vi "Periodic Tasks.vi"(8 "error in":errorcluster) -> ()   [LabVIEW 2014]
doc: "This VI runs in parallel to other tasks. It can contain as many user-defined periodic loops as you need. These can carry out PID or other sorts of timed response."
uses:
  <vilib>/Rock Robotics/WPI/DriverStation/WPI_DriverStationRobotMode2.ctl
  <vilib>/Rock Robotics/WPI/Solenoid/WPI_SolenoidValue.ctl
  <vilib>/Rock Robotics/WPI/RobotDrive/WPI_RobotDriveGetSetRefNum.vi
  <vilib>/Rock Robotics/WPI/Joystick/WPI_JoystickGetSetRefNum.vi
  Robot Global Data.vi
  <vilib>/Rock Robotics/Network Tables/SD Write Boolean.vi
  <vilib>/Rock Robotics/Network Tables/SD Write Number.vi
  <vilib>/Rock Robotics/WPI/Compressor/WPI_CompressorGetSetRefNum.vi
  Moose Code/Auto_Conf.vi
  <vilib>/Rock Robotics/WPI/Solenoid/WPI_SolenoidSetEnum.vi
  <vilib>/Rock Robotics/WPI/Solenoid/Deprecated/WPI_SolenoidSetBool.vi
panel:
  in  "Kpd":dbl=0.036
  in  "AllowZero":bool
  in  "ElevatorReset":bool
  out "GoatDetectorPhotoeye":bool
  out "D Contribution":dbl
  in  "Kd":dbl=0.075
  out "BottomOvertravel":bool=TRUE
  out "TopOvertravel":bool=TRUE
  out "ElevatorCurrent":dbl
  out "Voltage":dbl
  out "CurrentSum":dbl
  out "Motor Control":dbl(graph)
  in  "IZone":dbl=25.0
  out "Current":dbl
  out "Target":dbl
  out "PIDPhotoeye":bool
  in  "Kp":dbl=0.036
  in  "Ki":dbl=0.0005 step=0.0001
  out "Target vs. Actual":T1(graph)
  out "I Contribution":dbl
  out "P Contribution":dbl
  in  "Threshold":dbl=3.5
  out "In Position":bool
  out "EncoderLeft":dbl
  out "EncoderRight":dbl
  # "K Tune-torial: (copied from email)\n      Find a P gain that gets you close to your target without overshooting.  \nBased on that P gain value calculate the error at which your P starts to\ndecrease below full throttle.  Make your I cap equal to this error.  Make your\ninitial I gain very small (less than .1 say .0001).  The idea is to accumulate a \nvalue that is manageable. The Talon I accumulates every 1 millisecond so it\nis very easy to calculate the amount of time to get to full throttle.  An I gain\nof .001 will get you full throttle in about 1 second (assuming error never\nchanges).\n      The goal of this strategy is to make I perceivable while still allowing\nP to be the dominating component.  In position servo, I is only needed\nwhen P is not enough to get you to your target.  Once your P output is\nless than full throttle, I will start to kick in.  At first there will be a noticeable\ngap in throttle.  Throttle will decrease proportional to the error and then\nslowly ramp back up until the target is reached, this is useful in observing\nthe effect of I.  Slowly increase I and adjust the I zone until the throttle is \nalmost seamless."
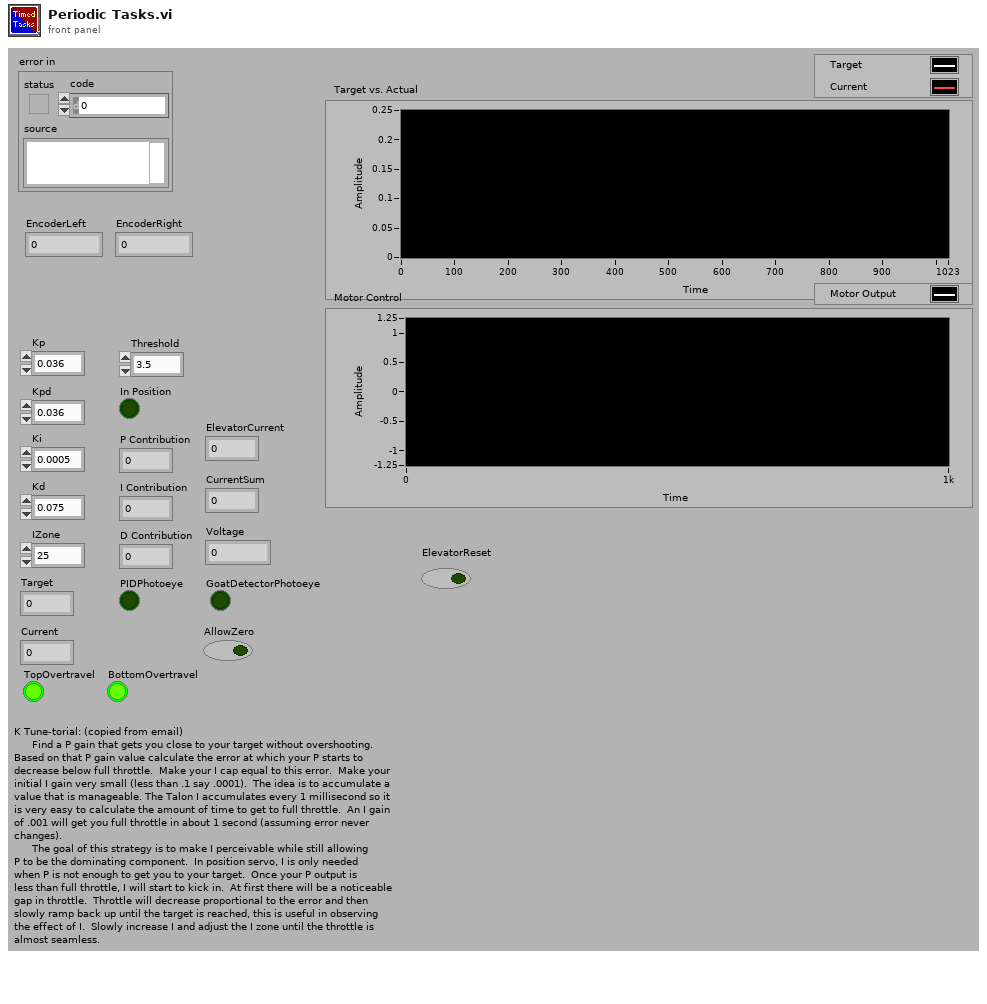
[diagram p1: front panel]
types:
  T1 = cluster{"[0]":dbl, "[1]":dbl, "[2]":dbl, "[3]":dbl, "[4]":dbl, "[5]":dbl, "[6]":dbl, "[7]":dbl, "[8]":dbl}
  T2 = enum16{"ResetForward", "ResetBack", "PIDControl", "ManualControl", "ZeroEncoderAndTarget", "AutoStack"}
  T3 = enum16{"Disabled", "Initialize", "CalcNewTarget", "Moving", "OpenArm", "CloseArm", "Reset"}
  T4 = typedef "WPI_EncoderDevRef.ctl" = cluster{"DevStatus":errorcluster, "EncoderIndex":T5, "CounterIndex":T6, "DistancePerCount":dbl, "Decoding Type":T7}
  T5 = typedef "FPGA_EncoderIdx.ctl" = enum8{"Enc 0", "Enc 1", "Enc 2", "Enc 3", "Enc 4", "Enc 5", "Enc 6", "Enc 7", "Invalid"}
  T6 = typedef "FPGA_CounterCtrSystemIndex.ctl" = enum8{"Ctr 0", "Ctr 1", "Ctr 2", "Ctr 3", "Ctr 4", "Ctr 5", "Ctr 6", "Ctr 7", "Invalid"}
  T7 = typedef "WPI_EncoderType.ctl" = enum16{"1x", "2x", "4x"}
  T8 = typedef "WPI_JoystickDevRef.ctl" = cluster{"Device":T9}
  T9 = typedef "WPI_JoystickDeviceEnum.ctl" = enum16{"USB 0", "USB 1", "USB 2", "USB 3", "USB 4", "USB 5"}
  T10 = typedef "WPI_SolenoidDevRef.ctl" = cluster{"DevStatus":errorcluster, "Pneumatics Control Module":u8, "Forward Solenoid Channel":T11, "Reverse Solenoid Channel":T11}
  T11 = typedef "WPI_SolenoidChannel.ctl" = enum8{"Solenoid 0", "Solenoid 1", "Solenoid 2", "Solenoid 3", "Solenoid 4", "Solenoid 5", "Solenoid 6", "Solenoid 7", "Invalid"}
  T12 = typedef "WPI_MotorControlDeviceRef.ctl" = cluster{"DeviceStatus":errorcluster, "Type":T13, "PWM":cluster{"Controller":T14, "PWM Channel":T15, "DeadBand":T16}, "CAN":cluster{"Device Number":u8, "Control Mode":T17, "Semaphore":T18, "Max Vout":dbl, "TalonSRX Control Mode":T19}, "Invert":bool, "TransformRef":T20, "InvTransformRef":T20}
  T13 = typedef "WPI_MotorControlType.ctl" = enum16{"PWM", "CAN", "CANTalonSRX"}
  T14 = typedef "FPGA_TypedefDigitalModule.ctl" = enum16{"Controller 1"}
  T15 = typedef "FPGA_DIOPWMChannel.ctl" = enum8{"PWM 0", "PWM 1", "PWM 2", "PWM 3", "PWM 4", "PWM 5", "PWM 6", "PWM 7", "PWM 8", "PWM 9", "PWM MXP 0", "PWM MXP 1", "PWM MXP 2", "PWM MXP 3", "PWM MXP 4", "PWM MXP 5", "PWM MXP 6", "PWM MXP 7", "PWM MXP 8", "PWM MXP 9", "Invalid"}
  T16 = typedef "WPI_PWMDeadband.ctl" = cluster{"Name":string, "maxPositivePwm":i32, "minPositivePwm":i32, "centerPwm":i32, "maxNegativePwm":i32, "minNegativePwm":i32, "angularRange":u16}
  T17 = typedef "WPI_CANJaguar_ControlMode.ctl" = enum8{"Percent VBus", "Current", "Speed", "Position", "Voltage"}
  T18 = typedef "Semaphore RefNum" = refnum<k1>
  T19 = typedef "WPI_CANTalonSRX_APIControlMode.ctl" = enum8{"Percent VBus", "Speed", "Position", "Slave", "Unchanged / Invalid"}
  T20 = typedef "WPI_PWMTransform_ConPane.ctl" = refnum<vi>
  T21 = typedef "WPI_RobotDriveDevRef.ctl" = cluster{"DevStatus":errorcluster, "Motors[]":T12[], "Square Inputs":bool, "Max Output":dbl}
  T22 = typedef "WPI_DigitalInputDevRef.ctl" = cluster{"DevStatus":errorcluster, "DIO Channel":T23, "Controller":T14}
  T23 = typedef "FPGA_DIOChannel.ctl" = enum8{"DIO 0", "DIO 1", "DIO 2", "DIO 3", "DIO 4", "DIO 5", "DIO 6", "DIO 7", "DIO 8", "DIO 9", "DIO MXP 0", "DIO MXP 1", "DIO MXP 2", "DIO MXP 3", "DIO MXP 4", "DIO MXP 5", "DIO MXP 6", "DIO MXP 7", "DIO MXP 8", "DIO MXP 9", "DIO MXP 10", "DIO MXP 11", "DIO MXP 12", "DIO MXP 13", "DIO MXP 14", "DIO MXP 15", "Invalid"}
  T24 = typedef "WPI_CompressorDevRef.ctl" = cluster{"DevStatus":errorcluster, "Pneumatics Control Module":u8}
  T25 = typedef "WPI_DriverStationRobotMode2.ctl" = enum16{"Autonomous Disabled", "Autonomous Enabled", "Teleop Disabled", "Teleop Enabled", "Disconnected", "Finish", "Test Disabled", "Test Enabled", "Emergency Stopped"}
  T26 = typedef "WPI_GyroDevRef.ctl" = cluster{"DevStatus":errorcluster, "Analog Module":T27, "Analog Channel":T28, "Offset":dbl, "Gain (VoltsPerDegree/Second)":dbl}
  T27 = typedef "FPGA_TypedefAnalogModule.ctl" = enum16{"Controller 1"}
  T28 = typedef "FPGA_AIChannel.ctl" = enum8{"AI 0", "AI 1", "AI 2", "AI 3", "AI MXP 0", "AI MXP 1", "AI MXP 2", "AI MXP 3", "Invalid"}
  T29 = typedef "WPI_SolenoidValue.ctl" = enum16{"Off", "On", "Forward", "Reverse"}
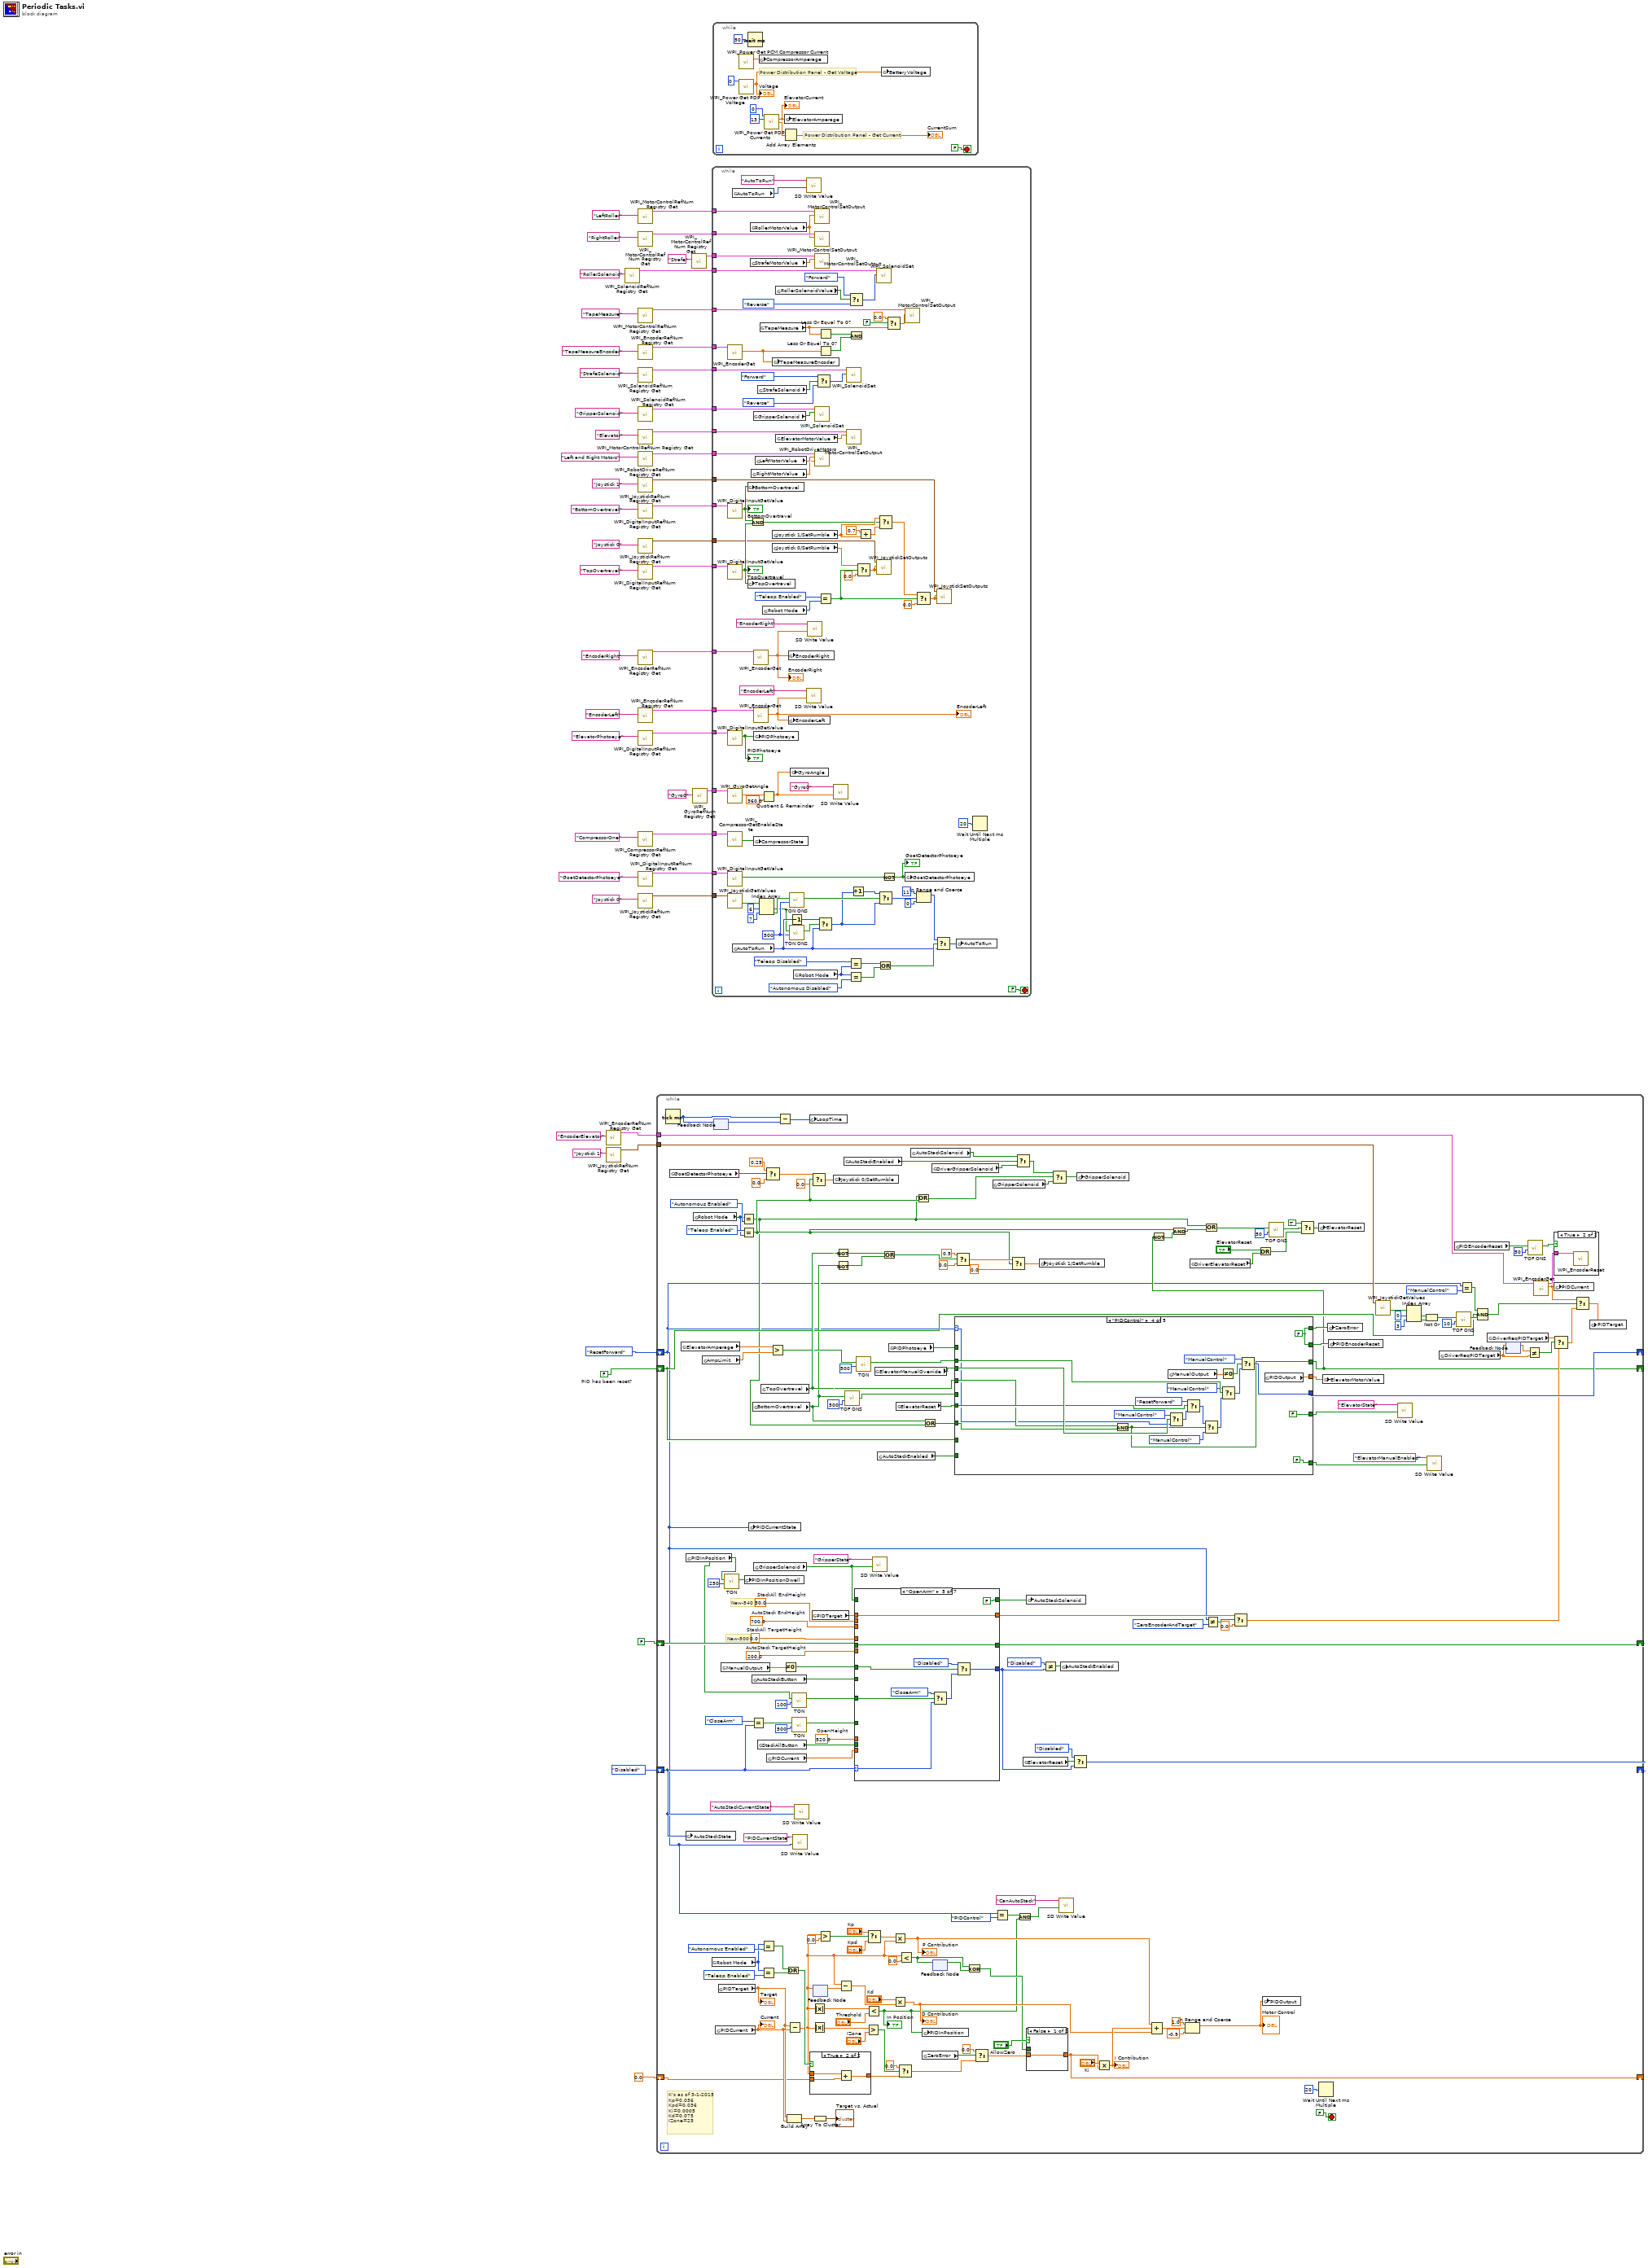
[diagram p0: block diagram]
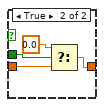
[diagram p4: hidden frame]
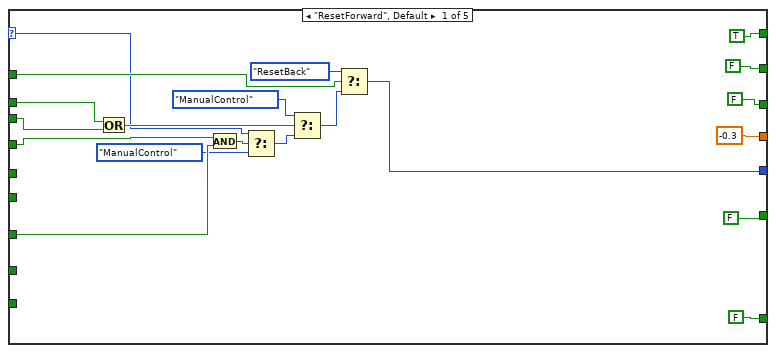
[diagram p5: hidden frame]
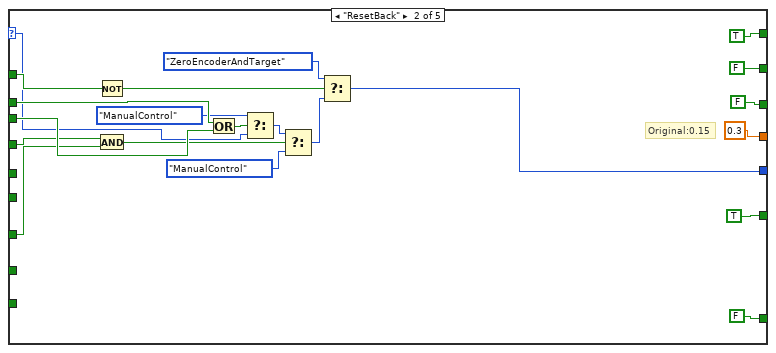
[diagram p6: hidden frame]
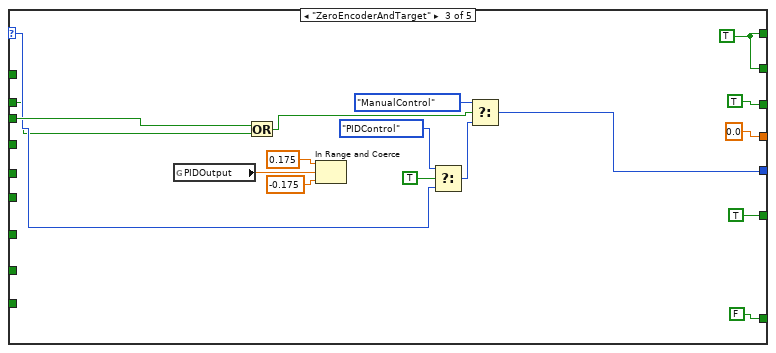
[diagram p7: hidden frame]
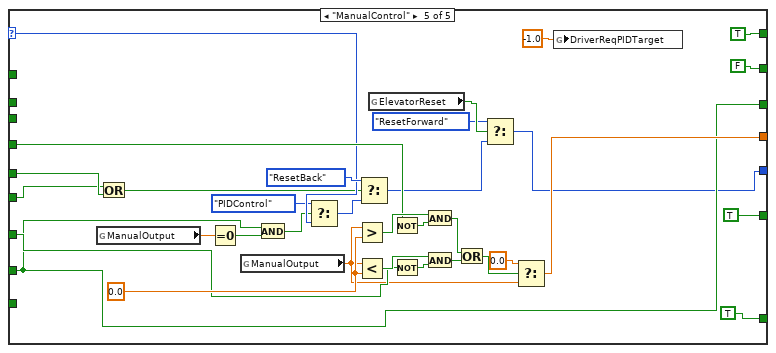
[diagram p8: hidden frame]
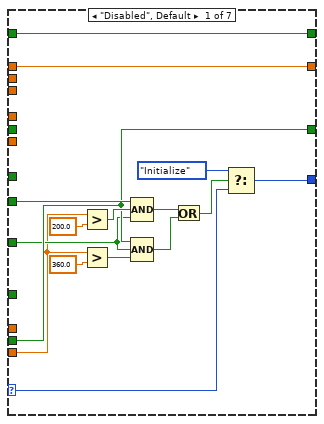
[diagram p9: hidden frame]
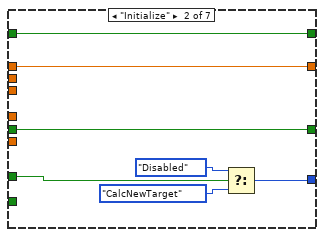
[diagram p10: hidden frame]
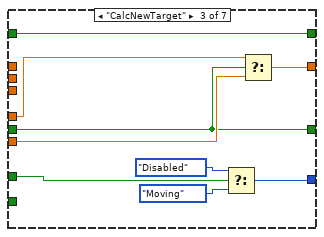
[diagram p11: hidden frame]
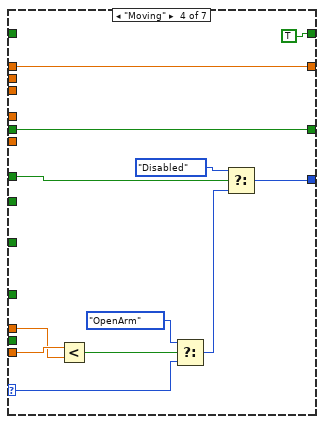
[diagram p12: hidden frame]
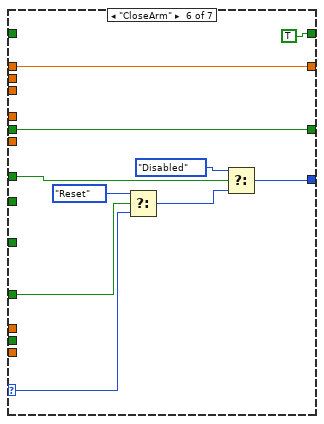
[diagram p13: hidden frame]
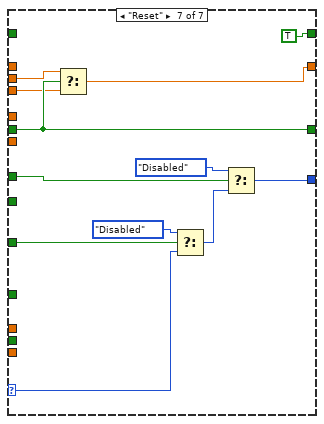
[diagram p14: hidden frame]
diagram:
  w20 = FALSE  # PID has been reset?
  n1 = call <vilib>:"WPI_EncoderRefNum Registry Get.vi"("refnum name"="EncoderElevator") -> ("EncoderDevRef"=w9:T4)  [unwired: 9 in, 1 out]
  n2 = call <vilib>:"WPI_JoystickRefNum Registry Get.vi"("refnum name"="Joystick 1") -> ("JoystickDevRef"=w7:T8)  [unwired: 9 in, 1 out]
  n3 = call <vilib>:"WPI_SolenoidRefNum Registry Get.vi"("refnum name"="RollerSolenoid") -> ("SolenoidDevRef"=w10:T10)  [unwired: 9 in, 1 out]
  n4 = call <vilib>:"WPI_MotorControlRefNum Registry Get.vi"("refnum name"="LeftRoller") -> ("MotorControlDevRef"=w13:T12)  [unwired: 9 in, 1 out]
  n5 = call <vilib>:"WPI_MotorControlRefNum Registry Get.vi"("refnum name"="RightRoller") -> ("MotorControlDevRef"=w12:T12)  [unwired: 9 in, 1 out]
  n6 = call <vilib>:"WPI_MotorControlRefNum Registry Get.vi"("refnum name"="TapeMeasure") -> ("MotorControlDevRef"=w4:T12)  [unwired: 9 in, 1 out]
  n7 = call <vilib>:"WPI_EncoderRefNum Registry Get.vi"("refnum name"="TapeMeasureEncoder") -> ("EncoderDevRef"=w1:T4)  [unwired: 9 in, 1 out]
  n8 = call <vilib>:"WPI_SolenoidRefNum Registry Get.vi"("refnum name"="StrafeSolenoid") -> ("SolenoidDevRef"=w16:T10)  [unwired: 9 in, 1 out]
  n9 = call <vilib>:"WPI_SolenoidRefNum Registry Get.vi"("refnum name"="GripperSolenoid") -> ("SolenoidDevRef"=w30:T10)  [unwired: 9 in, 1 out]
  n10 = call <vilib>:"WPI_MotorControlRefNum Registry Get.vi"("refnum name"="Elevator") -> ("MotorControlDevRef"=w46:T12)  [unwired: 9 in, 1 out]
  n11 = call <vilib>:"WPI_RobotDriveRefNum Registry Get.vi"("refnum name"="Left and Right Motors") -> ("RobotDriveDevRef"=w51:T21)  [unwired: 9 in, 1 out]
  n12 = call <vilib>:"WPI_JoystickRefNum Registry Get.vi"("refnum name"="Joystick 1") -> ("JoystickDevRef"=w27:T8)  [unwired: 1 in, 9 out]
  n13 = call <vilib>:"WPI_DigitalInputRefNum Registry Get.vi"("refnum name"="BottomOvertravel") -> ("DigitalInputDevRef"=w32:T22)  [unwired: 9 in, 1 out]
  n14 = call <vilib>:"WPI_JoystickRefNum Registry Get.vi"("refnum name"="Joystick 0") -> ("JoystickDevRef"=w26:T8)  [unwired: 1 in, 9 out]
  n15 = call <vilib>:"WPI_DigitalInputRefNum Registry Get.vi"("refnum name"="TopOvertravel") -> ("DigitalInputDevRef"=w34:T22)  [unwired: 9 in, 1 out]
  n16 = call <vilib>:"WPI_EncoderRefNum Registry Get.vi"("refnum name"="EncoderRight") -> ("EncoderDevRef"=w39:T4)  [unwired: 9 in, 1 out]
  n17 = call <vilib>:"WPI_EncoderRefNum Registry Get.vi"("refnum name"="EncoderLeft") -> ("EncoderDevRef"=w41:T4)  [unwired: 9 in, 1 out]
  n18 = call <vilib>:"WPI_DigitalInputRefNum Registry Get.vi"("refnum name"="ElevatorPhotoeye") -> ("DigitalInputDevRef"=w44:T22)  [unwired: 9 in, 1 out]
  n19 = call <vilib>:"WPI_CompressorRefNum Registry Get.vi"("refnum name"="CompressorOne") -> ("CompressorDevRef"=w5:T24)  [unwired: 9 in, 1 out]
  n20 = call <vilib>:"WPI_DigitalInputRefNum Registry Get.vi"("refnum name"="GoatDetectorPhotoeye") -> ("DigitalInputDevRef"=w24:T22)  [unwired: 9 in, 1 out]
  n21 = call <vilib>:"WPI_JoystickRefNum Registry Get.vi"("refnum name"="Joystick 0") -> ("JoystickDevRef"=w18:T8)  [unwired: 9 in, 1 out]
  n22 = while {
    shift-right: [w136] -> _
    shift-left: 0.0 -> [w65]
    shift-right: [w126] -> _
    shift-left: T3."Disabled" -> [w102]
    shift-right: [w202] -> _
    shift-left: FALSE -> [w204]
    shift-right: [w164] -> _
    shift-left: T2."ResetForward" -> [w56]
    shift-right: [w58] -> _
    shift-left: w20 -> [w109]
    tunnel: w9 -> [w96]
    tunnel: w7 -> [w92]
    stop <- FALSE stop-if-true
    w52 = 0.0  # StackAll TargetHeight
    w82 = 700.0  # AutoStack EndHeight
    w112 = 200.0  # AutoStack TargetHeight
    w113 = 30.0  # StackAll EndHeight
    w205 = 520.0  # OpenHeight
    # "New-500"
    # "New-540"
    # "K's as of 3-1-2015\nKp=0.036\nKpd=0.036\nKi=0.0005\nKd=0.075\nIZone=25"
    n23 = Tick Count (ms)() -> (millisecond timer value=w145:u32)
    n24 = global read "Robot Global Data.vi" "GoatDetectorPhotoeye"() -> (w197:bool)
    n25 = global read "Robot Global Data.vi" "ElevatorAmperage"() -> (w175:dbl)
    n26 = global write "Robot Global Data.vi" "AutoStackState"(w102) -> ()
    n27 = global read "Robot Global Data.vi" "PIDInPosition"() -> (w64:bool)
    n28 = global read "Robot Global Data.vi" "Robot Mode"() -> (w59:T25)
    n29 = global read "Robot Global Data.vi" "AmpLimit"() -> (w176:dbl)
    n30 = global read "Robot Global Data.vi" "Robot Mode"() -> (w69:T25)
    n31 = feedback-in #1(w145) -> ()
    n32 = feedback #1() -> (w144:u32)  [unwired: 1 in]
    n33 = global read "Robot Global Data.vi" "PIDCurrent"() -> (w220:dbl)
    "Current" <- w220
    n34 = global read "Robot Global Data.vi" "PIDTarget"() -> (w216:dbl)
    "Target" <- w216
    n35 = global read "Robot Global Data.vi" "ManualOutput"() -> (w111:dbl)
    n36 = call "TON.vi"("Delay (ms)"=u32 250, "Input"=w64) -> ("Output"=w105:bool)  [unwired: 9 in]
    n37 = Equal?(x=w59, y=WPI_DriverStationRobotMode2."Autonomous Enabled") -> (x = y?=w75:bool)
    n38 = Equal?(x=WPI_DriverStationRobotMode2."Teleop Enabled" ("y"), y=w59) -> (x = y?=w77:bool)
    n39 = global write "Robot Global Data.vi" "PIDInPositionDwell"(w105) -> ()
    n40 = global write "Robot Global Data.vi" "PIDCurrentState"(w56) -> ()
    n41 = Equal?(x=T3."CloseArm" ("t"), y=w102) -> (x = y?=w121:bool)
    n42 = global read "Robot Global Data.vi" "AutoStackButton"() -> (w206:bool)
    n43 = global read "Robot Global Data.vi" "BottomOvertravel"() -> (w84:bool)
    n44 = global read "Robot Global Data.vi" "GripperSolenoid"() -> (w87:bool)
    n45 = global read "Robot Global Data.vi" "StackAllButton"() -> (w208:bool)
    n46 = global read "Robot Global Data.vi" "TopOvertravel"() -> (w194:bool)
    n47 = Equal?(x=w69, y=WPI_DriverStationRobotMode2."Autonomous Enabled") -> (x = y?=w73:bool)
    n48 = Equal?(x=w69, y=WPI_DriverStationRobotMode2."Teleop Enabled") -> (x = y?=w72:bool)
    n49 = Select(t=0.25, s=w197, f=0.0) -> (s? t:f=w195:dbl)
    n50 = global read "Robot Global Data.vi" "PIDCurrent"() -> (w203:dbl)
    n51 = Greater?(x=w175, y=w176) -> (0:w177:bool)
    n52 = Subtract(x=w145, y=w144) -> (x-y=w143:u32)
    n53 = Not Equal To 0?(x=w111) -> (x != 0?=w110:bool)
    n54 = Or(x=w73, y=w72) -> (x .or. y?=w68:bool)
    n55 = Build Array(w216, w220) -> (w224:dbl[])
    n56 = Subtract(x=w216, y=w220) -> (x-y=w66:dbl)
    n57 = call "TON.vi"("Delay (ms)"=u32 100, "Input"=w64) -> ("Output"=w81:bool)  [unwired: 9 in]
    n58 = call "TON.vi"("Delay (ms)"=u32 500, "Input"=w121) -> ("Output"=w123:bool)  [unwired: 9 in]
    n59 = call-poly <vilib>:"SD Write Value.vi"("Numeric"=w56, "Name"="PIDCurrentState") -> ()  [unwired: 8 in, 2 out]
    n60 = call-poly <vilib>:"SD Write Value.vi"("Numeric"=w102, "Name"="AutoStackCurrentState") -> ()  [unwired: 8 in, 2 out]
    n61 = global write "Robot Global Data.vi" "LoopTime"(w143) -> ()
    n62 = case shown="True" w68 {
      tunnel: [w231 w234] -> w67
      tunnel: w66 -> [_ w233]
      tunnel: w65 -> [w231 w232]
      frame False {
      }
      frame True {
        n63 = Add(x=w233, y=w232) -> (x+y=w234:dbl)
      }
    }
    n64 = Select(t=w195, s=w77, f=0.0) -> (s? t:f=w180:dbl)
    n65 = global read "Robot Global Data.vi" "PIDTarget"() -> (w207:dbl)
    n66 = Absolute Value(x=w66) -> (abs(x)=w222:dbl)
    n67 = Absolute Value(x=w66) -> (abs(x)=w219:dbl)
    n68 = feedback-in #2(w66) -> ()
    n69 = feedback #2() -> (w215:dbl)  [unwired: 1 in]
    n70 = Array To Cluster(array=w224) -> (cluster=→"Target vs. Actual":T1)
    n71 = Greater?(x=w66, y=0.0) -> (0:w118:bool)
    n72 = global write "Robot Global Data.vi" "Joystick 0/SetRumble"(w180) -> ()
    n73 = Not(x=w194) -> (.not. x?=w192:bool)
    n74 = Not(x=w84) -> (.not. x?=w193:bool)
    n75 = Subtract(x=w66, y=w215) -> (x-y=w213:dbl)
    n76 = global read "Robot Global Data.vi" "AutoStackEnabled"() -> (w63:bool)
    n77 = call "TOF ONS.vi"("Delay (ms)"=u32 500, "Input"=w84) -> ("Output"=w107:bool)  [unwired: 9 in]
    n78 = case shown="\"OpenArm\"" w102 {
      selector: w102 -> [w370 _ _ w397 w405 w414 w428]
      tunnel: w205 -> [_ _ _ w387 _ _ _]
      tunnel: w112 -> [_ _ w384 _ _ _ _]
      tunnel: w206 -> [w361 _ _ _ _ _ _]
      tunnel: w207 -> [w355 w377 _ w394 w406 w416 _]
      tunnel: [w355 w377 w386 w394 w406 w416 w426] -> w161
      tunnel: w208 -> [w360 _ _ _ _ _ _]
      tunnel: [w360 w376 w379 w393 w408 w417 w425] -> w202
      tunnel: w204 -> [_ w376 w379 w393 w408 w417 w425]
      tunnel: [w366 w375 w385 TRUE FALSE ("Solenoid") TRUE ("Solenoid") TRUE ("Solenoid")] -> w209
      tunnel: w87 -> [w366 w375 w385 _ _ _ _]
      tunnel: [w368 w372 w381 w392 w402 w411 w422] -> w127
      tunnel: w81 -> [w358 _ _ _ w403 _ w429]
      tunnel: w203 -> [w356 _ _ w388 _ _ _]
      tunnel: w123 -> [_ _ _ _ _ w413 _]
      tunnel: w113 -> [_ _ _ _ _ _ w424]
      tunnel: w110 -> [_ w371 w380 w390 w399 w409 w421]
      tunnel: w82 -> [_ _ _ _ _ _ w419]
      tunnel: w52 -> [_ _ w378 _ _ _ _]
      frame "Disabled", Default {
        n79 = Greater?(x=w356, y=200.0) -> (0:w367:bool)
        n80 = Greater?(x=w356, y=360.0) -> (0:w357:bool)
        n81 = Compound Arithmetic op=AND(w361, w367, w358) -> (w364:bool)
        n82 = Compound Arithmetic op=AND(w360, w358, w357) -> (w362:bool)
        n83 = Or(x=w364, y=w362) -> (x .or. y?=w363:bool)
        n84 = Select(t=T3."Initialize", s=w363, f=w370) -> (s? t:f=w368:T3)
      }
      frame "Initialize" {
        n85 = Select(t=T3."Disabled", s=w371, f=T3."CalcNewTarget") -> (s? t:f=w372:T3)
      }
      frame "CalcNewTarget" {
        n86 = Select(t=T3."Disabled", s=w380, f=T3."Moving") -> (s? t:f=w381:T3)
        n87 = Select(t=w378, s=w379, f=w384) -> (s? t:f=w386:dbl)
      }
      frame "Moving" {
        n88 = Less?(x=w388, y=w387) -> (x < y?=w398:bool)
        n89 = Select(t=T3."OpenArm", s=w398, f=w397) -> (s? t:f=w391:T3)
        n90 = Select(t=T3."Disabled", s=w390, f=w391) -> (s? t:f=w392:T3)
      }
      frame "OpenArm" {
        n91 = Select(t=T3."CloseArm", s=w403, f=w405) -> (s? t:f=w401:T3)
        n92 = Select(t=T3."Disabled", s=w399, f=w401) -> (s? t:f=w402:T3)
      }
      frame "CloseArm" {
        n93 = Select(t=T3."Reset", s=w413, f=w414) -> (s? t:f=w410:T3)
        n94 = Select(t=T3."Disabled", s=w409, f=w410) -> (s? t:f=w411:T3)
      }
      frame "Reset" {
        n95 = Select(t=w424, s=w425, f=w419) -> (s? t:f=w426:dbl)
        n96 = Select(t=T3."Disabled", s=w429, f=w428) -> (s? t:f=w420:T3)
        n97 = Select(t=T3."Disabled", s=w421, f=w420) -> (s? t:f=w422:T3)
      }
    }
    n98 = call "TON.vi"("Delay (ms)"=u32 500, "Input"=w177) -> ("Output"=w178:bool)  [unwired: 9 in]
    n99 = Greater?(x=w219, y="IZone") -> (0:w155:bool)
    n100 = Select(t="Kp", s=w118, f="Kpd") -> (s? t:f=w117:dbl)
    n101 = Less?(x=w222, y="Threshold") -> (x < y?=w54:bool)
    "In Position" <- w54
    n102 = call-poly <vilib>:"SD Write Value.vi"("Boolean"=w87, "Name"="GripperState") -> ()  [unwired: 8 in, 2 out]
    n103 = global read "Robot Global Data.vi" "ElevatorManualOverride"() -> (w169:bool)
    n104 = global read "Robot Global Data.vi" "AutoStackEnabled"() -> (w62:bool)
    n105 = Or(x=w192, y=w193) -> (x .or. y?=w190:bool)
    n106 = global read "Robot Global Data.vi" "PIDPhotoeye"() -> (w168:bool)
    n107 = Multiply(x=w117, y=w66) -> (x*y=w156:dbl)
    "P Contribution" <- w156
    n108 = Multiply(x="Kd", y=w213) -> (x*y=w212:dbl)
    "D Contribution" <- w212
    n109 = global read "Robot Global Data.vi" "ElevatorReset"() -> (w170:bool)
    n110 = Select(t=0.0, s=w155, f=w67) -> (s? t:f=w130:dbl)
    n111 = Less?(x=w66, y=0.0) -> (x < y?=w139:bool)
    n112 = global read "Robot Global Data.vi" "AutoStackSolenoid"() -> (w184:bool)
    n113 = Or(x=w75, y=w77) -> (x .or. y?=w186:bool)
    n114 = global write "Robot Global Data.vi" "PIDInPosition"(w54) -> ()
    n115 = global read "Robot Global Data.vi" "ZeroError"() -> (w132:bool)
    n116 = Or(x=w84, y=w75) -> (x .or. y?=w83:bool)
    n117 = global read "Robot Global Data.vi" "DriverGripperSolenoid"() -> (w183:bool)
    n118 = feedback-in #3(w139) -> ()
    n119 = feedback #3() -> (w138:bool)  [unwired: 1 in]
    n120 = case shown="\"PIDControl\"" w56 {
      selector: w56 -> [w242 w263 w293 w302 w334]
      tunnel: [-0.3 0.3 0.0 ("ManualOutput") w301 w353] -> w167
      tunnel: [w244 w264 w298 w306 w323] -> w164
      tunnel: w168 -> [w259 w280 _ _ _]
      tunnel: w169 -> [w246 w278 w297 w321 _]
      tunnel: w170 -> [_ _ _ w320 w329]
      tunnel: [FALSE ("PIDEncoderReset") FALSE ("PIDEncoderReset") w289 w318 FALSE ("PIDEncoderReset")] -> w174
      tunnel: [TRUE ("PIDEncoderReset") TRUE ("PIDEncoderReset") w289 w318 TRUE ("PIDEncoderReset")] -> w79
      tunnel: w194 -> [w256 w274 _ w315 w351]
      tunnel: w83 -> [w255 w273 _ w314 w345]
      tunnel: w178 -> [w248 w270 w287 w313 _]
      tunnel: [FALSE ("PIDEncoderReset") FALSE ("PIDEncoderReset") FALSE ("PIDEncoderReset") FALSE ("PIDEncoderReset") TRUE ("PIDEncoderReset")] -> w151
      tunnel: w62 -> [_ _ _ _ _]
      tunnel: w109 -> [_ _ _ _ w331]
      tunnel: [FALSE FALSE TRUE w299 w331] -> w58
      tunnel: w107 -> [_ _ _ _ w330]
      tunnel: [FALSE ("PIDEncoderReset") TRUE ("PIDEncoderReset") TRUE ("PIDEncoderReset") FALSE ("PIDEncoderReset") TRUE ("PIDEncoderReset")] -> w85
      frame "ResetForward", Default {
        n121 = Or(x=w248, y=w246) -> (x .or. y?=w247:bool)
        n122 = And(x=w256, y=w255) -> (x .and. y?=w257:bool)
        n123 = Select(t=w242, s=w257, f=T2."ManualControl") -> (s? t:f=w252:T2)
        n124 = Select(t=T2."ManualControl", s=w247, f=w252) -> (s? t:f=w243:T2)
        n125 = Select(t=T2."ResetBack", s=w259, f=w243) -> (s? t:f=w244:T2)
      }
      frame "ResetBack" {
        # "Original:0.15"
        n126 = Not(x=w280) -> (.not. x?=w279:bool)
        n127 = And(x=w274, y=w273) -> (x .and. y?=w276:bool)
        n128 = Or(x=w270, y=w278) -> (x .or. y?=w271:bool)
        n129 = Select(t=T2."ManualControl", s=w271, f=w263) -> (s? t:f=w275:T2)
        n130 = Select(t=w275, s=w276, f=T2."ManualControl") -> (s? t:f=w262:T2)
        n131 = Select(t=T2."ZeroEncoderAndTarget", s=w279, f=w262) -> (s? t:f=w264:T2)
      }
      frame "ZeroEncoderAndTarget" {
        w289 = TRUE ("PIDEncoderReset")
        n132 = global read "Robot Global Data.vi" "PIDOutput"() -> (w292:dbl)
        n133 = Or(x=w297, y=w287) -> (x .or. y?=w288:bool)
        n134 = In Range and Coerce(upper limit=0.175, x=w292, lower limit=-0.175) -> ()  [unwired: 2 out]
        n135 = Select(t=T2."PIDControl", s=TRUE, f=w293) -> (s? t:f=w295:T2)
        n136 = Select(t=T2."ManualControl", s=w288, f=w295) -> (s? t:f=w298:T2)
      }
      frame "PIDControl" {
        w318 = FALSE ("PIDEncoderReset")
        n137 = And(x=w315, y=w314) -> (x .and. y?=w299:bool)
        n138 = global read "Robot Global Data.vi" "ManualOutput"() -> (w304:dbl)
        n139 = Select(t=T2."ManualControl", s=w321, f=w302) -> (s? t:f=w319:T2)
        n140 = Select(t=T2."ResetForward", s=w320, f=w319) -> (s? t:f=w316:T2)
        n141 = Select(t=w316, s=w299, f=T2."ManualControl") -> (s? t:f=w317:T2)
        n142 = Not Equal To 0?(x=w304) -> (x != 0?=w303:bool)
        n143 = Select(t=T2."ManualControl", s=w313, f=w317) -> (s? t:f=w307:T2)
        n144 = Select(t=T2."ManualControl", s=w303, f=w307) -> (s? t:f=w306:T2)
        n145 = global read "Robot Global Data.vi" "PIDOutput"() -> (w301:dbl)
      }
      frame "ManualControl" {
        w347 = 0.0 ("y")
        n146 = global read "Robot Global Data.vi" "ManualOutput"() -> (w337:dbl)
        n147 = Or(x=w329, y=w330) -> (x .or. y?=w328:bool)
        n148 = Equal To 0?(x=w337) -> (x = 0?=w336:bool)
        n149 = global read "Robot Global Data.vi" "ManualOutput"() -> (w343:dbl)
        n150 = And(x=w331, y=w336) -> (x .and. y?=w332:bool)
        n151 = Select(t=T2."PIDControl", s=w332, f=w334) -> (s? t:f=w335:T2)
        n152 = Greater?(x=w343, y=w347) -> (0:w352:bool)
        n153 = Less?(x=w343, y=w347) -> (x < y?=w346:bool)
        n154 = Select(t=T2."ResetBack", s=w328, f=w335) -> (s? t:f=w324:T2)
        n155 = global read "Robot Global Data.vi" "ElevatorReset"() -> (w325:bool)
        n156 = Not(x=w351) -> (.not. x?=w341:bool)
        n157 = Not(x=w345) -> (.not. x?=w342:bool)
        n158 = And(x=w352, y=w341) -> (x .and. y?=w349:bool)
        n159 = And(x=w346, y=w342) -> (x .and. y?=w344:bool)
        n160 = Or(x=w349, y=w344) -> (x .or. y?=w348:bool)
        n161 = Select(t=T2."ResetForward", s=w325, f=w324) -> (s? t:f=w323:T2)
        n162 = Select(t=0.0, s=w348, f=w343) -> (s? t:f=w353:dbl)
        n163 = global write "Robot Global Data.vi" "DriverReqPIDTarget"(-1.0 ("DriverReqPIDTarget")) -> ()
      }
    }
    n164 = Select(t=0.5, s=w190, f=0.0) -> (s? t:f=w189:dbl)
    n165 = Exclusive Or(1:w138, 2:w139) -> (0:w135:bool)
    n166 = Select(t=0.0, s=w132, f=w130) -> (s? t:f=w133:dbl)
    n167 = global read "Robot Global Data.vi" "GripperSolenoid"() -> (w187:bool)
    n168 = Equal?(x=w56, y=T2."PIDControl") -> (x = y?=w55:bool)
    n169 = Select(t=w189, s=w77, f=0.0) -> (s? t:f=w181:dbl)
    n170 = Select(t=w184, s=w63, f=w183) -> (s? t:f=w185:bool)
    n171 = And(x=w55, y=w54) -> (x .and. y?=w53:bool)
    n172 = global read "Robot Global Data.vi" "ElevatorReset"() -> (w125:bool)
    n173 = global write "Robot Global Data.vi" "AutoStackSolenoid"(w209) -> ()
    n174 = case shown="False" "AllowZero" {
      tunnel: [w236 w240] -> w136
      tunnel: w135 -> [_ w239]
      tunnel: w133 -> [w236 w238]
      frame False {
      }
      frame True {
        n175 = Select(t=0.0, s=w239, f=w238) -> (s? t:f=w240:dbl)
      }
    }
    n176 = global write "Robot Global Data.vi" "Joystick 1/SetRumble"(w181) -> ()
    n177 = Not Equal?(x=T3."Disabled", y=w127) -> (x != y?=w211:bool)
    n178 = Select(t=w185, s=w186, f=w187) -> (s? t:f=w114:bool)
    n179 = call-poly <vilib>:"SD Write Value.vi"("Boolean"=w53, "Name"="CanAutoStack") -> ()  [unwired: 8 in, 2 out]
    n180 = global write "Robot Global Data.vi" "AutoStackEnabled"(w211) -> ()
    n181 = Select(t=T3."Disabled", s=w125, f=w127) -> (s? t:f=w126:T3)
    n182 = global write "Robot Global Data.vi" "GripperSolenoid"(w114) -> ()
    n183 = Multiply(x="Ki", y=w136) -> (x*y=w229:dbl)
    "I Contribution" <- w229
    n184 = Not(x=w58) -> (.not. x?=w78:bool)
    n185 = Compound Arithmetic op=ADD(w156, w229, w212) -> (w225:dbl)
    n186 = And(x=w77, y=w78) -> (x .and. y?=w76:bool)
    n187 = In Range and Coerce(upper limit=1.0, x=w225, lower limit=-0.9) -> (coerced(x)=w217:dbl)  [unwired: 1 out]
    "Motor Control" <- w217
    n188 = global read "Robot Global Data.vi" "DriverElevatorReset"() -> (w199:bool)
    n189 = Or(x=w75, y=w76) -> (x .or. y?=w74:bool)
    n190 = Not Equal?(x=w56, y=T2."ZeroEncoderAndTarget") -> (x != y?=w163:bool)
    n191 = Select(t=w161, s=w163, f=0.0) -> (s? t:f=w147:dbl)
    n192 = Or(x="ElevatorReset", y=w199) -> (x .or. y?=w201:bool)
    n193 = global write "Robot Global Data.vi" "PIDOutput"(w217) -> ()
    n194 = call "TOF ONS.vi"("Delay (ms)"=u32 50, "Input"=w74) -> ("Output"=w171:bool)  [unwired: 9 in]
    n195 = Select(t=TRUE, s=w171, f=w201) -> (s? t:f=w173:bool)
    n196 = global write "Robot Global Data.vi" "ElevatorReset"(w173) -> ()
    n197 = Wait Until Next ms Multiple(millisecond multiple=u32 20) -> ()  [unwired: 1 out]
    n198 = global write "Robot Global Data.vi" "ElevatorMotorValue"(w167) -> ()
    n199 = global write "Robot Global Data.vi" "ZeroError"(w79) -> ()
    n200 = global write "Robot Global Data.vi" "PIDEncoderReset"(w174) -> ()
    n201 = call <vilib>:"WPI_JoystickGetValues.vi"("JoystickDevRef"=w92) -> ("Buttons"=w95:bool[])  [unwired: 6 in, 4 out]
    n202 = call-poly <vilib>:"SD Write Value.vi"("Boolean"=w85, "Name"="ElevatorState") -> ()  [unwired: 8 in, 2 out]
    n203 = Index Array(array=w95, index #1=0 ("index"), index #2=3 ("index")) -> (element #1=w91:bool, element #2=w90:bool)
    n204 = Not Or(1:w90, 2:w91) -> (0:w89:bool)
    n205 = call-poly <vilib>:"SD Write Value.vi"("Boolean"=w151, "Name"="ElevatorManualEnabled") -> ()  [unwired: 8 in, 2 out]
    n206 = global read "Robot Global Data.vi" "DriverReqPIDTarget"() -> (w142:dbl)
    n207 = global read "Robot Global Data.vi" "PIDEncoderReset"() -> (w100:bool)
    n208 = call "TOF ONS.vi"("Delay (ms)"=u32 10, "Input"=w89) -> ("Output"=w153:bool)  [unwired: 9 in]
    n209 = Equal?(x=w56, y=T2."ManualControl") -> (x = y?=w157:bool)
    n210 = Compound Arithmetic op=AND(w157, w109, w153) -> (w152:bool)
    n211 = global read "Robot Global Data.vi" "DriverReqPIDTarget"() -> (w148:dbl)
    n212 = feedback-in #4(w142) -> ()
    n213 = feedback #4() -> (w141:dbl)  [unwired: 1 in]
    n214 = Not Equal?(x=w141, y=w142) -> (x != y?=w149:bool)
    n215 = call "TOF ONS.vi"("Delay (ms)"=u32 50, "Input"=w100) -> ("Output"=w99:bool)  [unwired: 9 in]
    n216 = call <vilib>:"WPI_EncoderGet.vi"("EncoderDevRef"=w96) -> ("Distance"=w97:dbl, "EncoderDevRef"=w101:T4)  [unwired: 5 in, 4 out]
    n217 = Select(t=w148, s=w149, f=w147) -> (s? t:f=w146:dbl)
    n218 = case shown="True" w99 {
      tunnel: w101 -> [_ w235]
      frame False {
      }
      frame True {
        n219 = call <vilib>:"WPI_EncoderReset.vi"("EncoderDevRef"=w235) -> ()  [unwired: 9 in, 2 out]
      }
    }
    n220 = global write "Robot Global Data.vi" "PIDCurrent"(w97) -> ()
    n221 = Select(t=w97, s=w152, f=w146) -> (s? t:f=w159:dbl)
    n222 = global write "Robot Global Data.vi" "PIDTarget"(w159) -> ()
  }
  n223 = call <vilib>:"WPI_MotorControlRefNum Registry Get.vi"("refnum name"="Strafe") -> ("MotorControlDevRef"=w48:T12)  [unwired: 9 in, 1 out]
  n224 = call <vilib>:"WPI_GyroRefNum Registry Get.vi"("refnum name"="Gyro0") -> ("GyroDevRef"=w37:T26)  [unwired: 9 in, 1 out]
  n225 = while {
    tunnel: w51 -> [w525]
    tunnel: w48 -> [w524]
    tunnel: w46 -> [w519]
    tunnel: w44 -> [w518]
    tunnel: w41 -> [w517]
    tunnel: w39 -> [w516]
    tunnel: w37 -> [w514]
    tunnel: w34 -> [w511]
    tunnel: w32 -> [w510]
    tunnel: w30 -> [w509]
    tunnel: w27 -> [w466]
    tunnel: w26 -> [w458]
    tunnel: w24 -> [w501]
    tunnel: w18 -> [w474]
    tunnel: w16 -> [w473]
    tunnel: w13 -> [w456]
    tunnel: w12 -> [w455]
    tunnel: w10 -> [w454]
    tunnel: w5 -> [w448]
    tunnel: w4 -> [w446]
    tunnel: w1 -> [w444]
    stop <- FALSE stop-if-true
    w481 = u32 500 ("Delay (ms)")
    n226 = call <vilib>:"WPI_EncoderGet.vi"("EncoderDevRef"=w444) -> ("Distance"=w431:dbl)  [unwired: 5 in, 5 out]
    n227 = call <vilib>:"WPI_DigitalInputGetValue.vi"("DigitalInputDevRef"=w510) -> ("Value"=w504:bool)  [unwired: 8 in, 2 out]
    "BottomOvertravel" <- w504
    n228 = call <vilib>:"WPI_DigitalInputGetValue.vi"("DigitalInputDevRef"=w511) -> ("Value"=w505:bool)  [unwired: 8 in, 2 out]
    "TopOvertravel" <- w505
    n229 = call <vilib>:"WPI_DigitalInputGetValue.vi"("DigitalInputDevRef"=w518) -> ("Value"=w515:bool)  [unwired: 8 in, 2 out]
    "PIDPhotoeye" <- w515
    n230 = call <vilib>:"WPI_GyroGetAngle.vi"("GyroDevRef"=w514) -> ("Angle"=w513:dbl)  [unwired: 7 in, 3 out]
    n231 = call <vilib>:"WPI_CompressorGetEnableState.vi"("CompressorDevRef"=w448) -> ("Compressor Running"=w447:bool)  [unwired: 7 in, 3 out]
    n232 = call <vilib>:"WPI_DigitalInputGetValue.vi"("DigitalInputDevRef"=w501) -> ("Value"=w502:bool)  [unwired: 8 in, 2 out]
    n233 = call <vilib>:"WPI_JoystickGetValues.vi"("JoystickDevRef"=w474) -> ("Buttons"=w478:bool[])  [unwired: 6 in, 4 out]
    n234 = global read "Auto_Conf.vi" "AutoToRun"() -> (w486:u8)
    n235 = global read "Auto_Conf.vi" "AutoToRun"() -> (w499:u8)
    n236 = global write "Robot Global Data.vi" "BottomOvertravel"(w504) -> ()
    n237 = global write "Robot Global Data.vi" "TopOvertravel"(w505) -> ()
    n238 = global read "Robot Global Data.vi" "RollerMotorValue"() -> (w433:dbl)
    n239 = global read "Robot Global Data.vi" "StrafeMotorValue"() -> (w523:dbl)
    n240 = And(x=w504, y=w505) -> (x .and. y?=w503:bool)
    n241 = global read "Robot Global Data.vi" "RightMotorValue"() -> (w521:dbl)
    n242 = global read "Robot Global Data.vi" "GripperSolenoid"() -> (w472:bool)
    n243 = call <vilib>:"WPI_EncoderGet.vi"("EncoderDevRef"=w516) -> ("Distance"=w437:dbl)  [unwired: 5 in, 5 out]
    "EncoderRight" <- w437
    n244 = call <vilib>:"WPI_EncoderGet.vi"("EncoderDevRef"=w517) -> ("Distance"=w435:dbl)  [unwired: 5 in, 5 out]
    "EncoderLeft" <- w435
    n245 = global write "Robot Global Data.vi" "PIDPhotoeye"(w515) -> ()
    n246 = global write "Robot Global Data.vi" "CompressorState"(w447) -> ()
    n247 = global read "Robot Global Data.vi" "LeftMotorValue"() -> (w522:dbl)
    n248 = global read "Robot Global Data.vi" "StrafeSolenoid"() -> (w470:bool)
    n249 = Index Array(array=w478, index #1=6 ("index"), index #2=7 ("index")) -> (element #1=w479:bool, element #2=w480:bool)
    n250 = global read "Robot Global Data.vi" "TapeMeasure"() -> (w439:dbl)
    n251 = Quotient & Remainder(x=w513, y=360.0) -> (x-y*floor(x/y)=w449:dbl)  [unwired: 1 out]
    n252 = global read "Robot Global Data.vi" "Robot Mode"() -> (w468:T25)
    n253 = global read "Robot Global Data.vi" "Joystick 1/SetRumble"() -> (w506:dbl)
    n254 = global read "Robot Global Data.vi" "Joystick 0/SetRumble"() -> (w459:dbl)
    n255 = global write "Robot Global Data.vi" "TapeMeasureEncoder"(w431) -> ()
    n256 = global read "Robot Global Data.vi" "RollerSolenoidValue"() -> (w445:bool)
    n257 = global read "Robot Global Data.vi" "ElevatorMotorValue"() -> (w520:dbl)
    n258 = global write "Robot Global Data.vi" "EncoderRight"(w437) -> ()
    n259 = global write "Robot Global Data.vi" "EncoderLeft"(w435) -> ()
    n260 = call "TON ONS.vi"("Delay (ms)"=w481, "Input"=w480) -> ("Output 2"=w488:bool)  [unwired: 9 in]
    n261 = call "TON ONS.vi"("Delay (ms)"=w481, "Input"=w479) -> ("Output 2"=w487:bool)  [unwired: 9 in]
    n262 = Decrement(x=w499) -> (x-1=w484:u8)
    n263 = global write "Robot Global Data.vi" "GyroAngle"(w449) -> ()
    n264 = global read "Robot Global Data.vi" "Robot Mode"() -> (w493:T25)
    n265 = call-poly <vilib>:"SD Write Value.vi"("Numeric"=w486, "Name"="AutoToRun") -> ()  [unwired: 8 in, 2 out]
    n266 = call-poly <vilib>:"SD Write Value.vi"("Numeric"=w435, "Name"="EncoderLeft") -> ()  [unwired: 8 in, 2 out]
    n267 = call-poly <vilib>:"SD Write Value.vi"("Numeric"=w437, "Name"="EncoderRight") -> ()  [unwired: 8 in, 2 out]
    n268 = call <vilib>:"WPI_MotorControlSetOutput.vi"("Output"=w433, "MotorControlDevRef"=w456) -> ()  [unwired: 7 in, 3 out]
    n269 = call <vilib>:"WPI_MotorControlSetOutput.vi"("Output"=w433, "MotorControlDevRef"=w455) -> ()  [unwired: 7 in, 3 out]
    n270 = call <vilib>:"WPI_MotorControlSetOutput.vi"("Output"=w523, "MotorControlDevRef"=w524) -> ()  [unwired: 7 in, 3 out]
    n271 = call-poly <vilib>:"WPI_SolenoidSet.vi"("Value"=w472, "SolenoidDevRef"=w509) -> ()  [unwired: 8 in, 2 out]
    n272 = call <vilib>:"WPI_RobotDriveMotors.vi"("RightSpeed"=w521, "LeftSpeed"=w522, "RobotDriveDevRef"=w525) -> ()  [unwired: 6 in, 3 out]
    n273 = Select(t=WPI_SolenoidValue."Forward" ("Value"), s=w470, f=WPI_SolenoidValue."Reverse") -> (s? t:f=w471:T29)
    n274 = Select(t=w484, s=w487, f=w499) -> (s? t:f=w483:u8)
    n275 = Less Or Equal To 0?(x=w439) -> (x <= 0?=w441:bool)
    n276 = Less Or Equal To 0?(x=w431) -> (x <= 0?=w443:bool)
    n277 = Equal?(x=WPI_DriverStationRobotMode2."Teleop Enabled" ("y"), y=w468) -> (x = y?=w461:bool)
    n278 = call-poly <vilib>:"SD Write Value.vi"("Numeric"=w449, "Name"="Gyro0") -> ()  [unwired: 8 in, 2 out]
    n279 = call-poly <vilib>:"WPI_SolenoidSet.vi"("Value"=w471, "SolenoidDevRef"=w473) -> ()  [unwired: 8 in, 2 out]
    n280 = call <vilib>:"WPI_MotorControlSetOutput.vi"("Output"=w520, "MotorControlDevRef"=w519) -> ()  [unwired: 7 in, 3 out]
    n281 = Select(t=WPI_SolenoidValue."Forward" ("Value"), s=w445, f=WPI_SolenoidValue."Reverse") -> (s? t:f=w452:T29)
    n282 = Equal?(x=WPI_DriverStationRobotMode2."Teleop Disabled" ("y"), y=w493) -> (x = y?=w496:bool)
    n283 = Equal?(x=w493, y=WPI_DriverStationRobotMode2."Autonomous Disabled") -> (x = y?=w495:bool)
    n284 = And(x=w441, y=w443) -> ()  [unwired: 1 out]
    n285 = Increment(x=w483) -> (x+1=w482:u8)
    n286 = Select(t=w459, s=w461, f=0.0) -> (s? t:f=w460:dbl)
    n287 = Add(x=0.7, y=w506) -> (x+y=w508:dbl)
    n288 = call-poly <vilib>:"WPI_SolenoidSet.vi"("Value"=w452, "SolenoidDevRef"=w454) -> ()  [unwired: 8 in, 2 out]
    n289 = call <vilib>:"WPI_JoystickSetOutputs.vi"("Right Rumble"=w460, "Left Rumble"=w460, "JoystickDevRef"=w458) -> ()  [unwired: 7 in, 2 out]
    n290 = Select(t=w506, s=w503, f=w508) -> (s? t:f=w465:dbl)
    n291 = Select(t=w482, s=w488, f=w483) -> (s? t:f=w489:u8)
    n292 = Or(x=w496, y=w495) -> (x .or. y?=w500:bool)
    n293 = Not(x=w502) -> (.not. x?=w434:bool)
    "GoatDetectorPhotoeye" <- w434
    n294 = Select(t=0.0, s=FALSE, f=w439) -> (s? t:f=w440:dbl)
    n295 = call <vilib>:"WPI_MotorControlSetOutput.vi"("Output"=w440, "MotorControlDevRef"=w446) -> ()  [unwired: 7 in, 3 out]
    n296 = global write "Robot Global Data.vi" "GoatDetectorPhotoeye"(w434) -> ()
    n297 = Select(t=w465, s=w461, f=0.0) -> (s? t:f=w463:dbl)
    n298 = In Range and Coerce(upper limit=u8 11, x=w489, lower limit=u8 0) -> (coerced(x)=w498:u8)  [unwired: 1 out]
    n299 = Select(t=w498, s=w500, f=w499) -> (s? t:f=w497:u8)
    n300 = call <vilib>:"WPI_JoystickSetOutputs.vi"("Right Rumble"=w463, "Left Rumble"=w463, "JoystickDevRef"=w466) -> ()  [unwired: 7 in, 2 out]
    n301 = global write "Auto_Conf.vi" "AutoToRun"(w497) -> ()
    n302 = Wait Until Next ms Multiple(millisecond multiple=u32 20 ("milliseconds to wait")) -> ()  [unwired: 1 out]
  }
  n303 = while {
    stop <- FALSE stop-if-true
    # "Power Distribution Panel - Get Voltage"
    # "Power Distribution Panel - Get Current"
    n304 = call <vilib>:"WPI_Power Get PCM Compressor Current.vi"() -> ("current (A)"=w528:dbl)  [unwired: 14 in, 1 out]
    n305 = call <vilib>:"WPI_Power Get PDP Voltage.vi"("Power Distribution Panel (0)"=u8 0) -> ("voltage (V)"=w529:dbl)  [unwired: 13 in, 1 out]
    "Voltage" <- w529
    n306 = Wait (ms)(milliseconds to wait=u32 50) -> ()  [unwired: 1 out]
    n307 = global write "Robot Global Data.vi" "CompressorAmperage"(w528) -> ()
    n308 = call <vilib>:"WPI_Power Get PDP Currents.vi"("Power Distribution Panel (0)"=u8 0, "PDP Channel"=13) -> ("current (A)"=w530:dbl, "all currents (A)"=w535:dbl[])  [unwired: 11 in, 1 out]
    "ElevatorCurrent" <- w530
    n309 = Add Array Elements(numeric array=w535) -> (sum=→"CurrentSum":dbl)
    n310 = global write "Robot Global Data.vi" "ElevatorAmperage"(w530) -> ()
    n311 = global write "Robot Global Data.vi" "BatteryVoltage"(w529) -> ()
  }
